vi "Render.vi"(8 "error in (no error)":errorcluster, 10 "String in":string, 11 "FencedCodeBlock in":refnum<class "FencedCodeBlock.lvclass">) -> (0 "error out":errorcluster, 2 "String out":string, 3 "FencedCodeBlock out":refnum<class "FencedCodeBlock.lvclass">)   [LabVIEW 2021, in "LvMarkdown.lvlib" / "FencedCodeBlock.lvclass"]
uses:
  FencedCodeBlock.lvclass
  C:/GitHub/LvMarkdown/src/LvMarkdown/Markdown.lvclass
  FencedCodeBlock.lvclass/FencedCodeBlock.ctl
  GetLanguage.vi
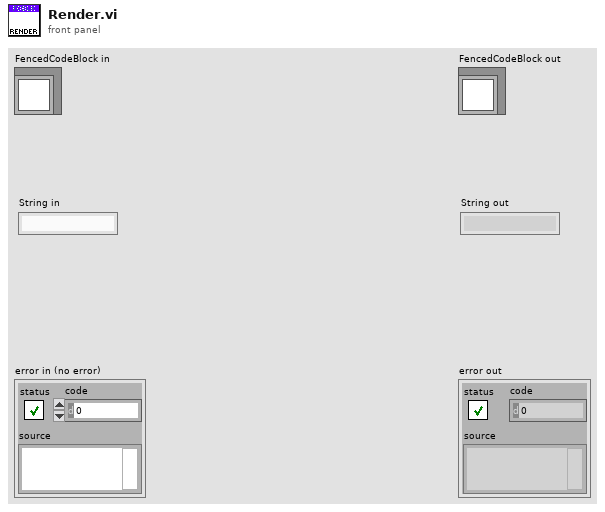
[diagram p1: front panel]
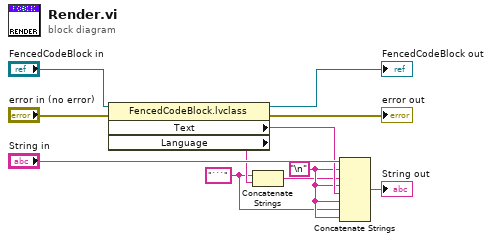
[diagram p0: block diagram]
diagram:
  w1 = "```" ("string")
  w9 = "\n"
  n1 = property class="FencedCodeBlock.lvclass"(reference="FencedCodeBlock in", error in="error in (no error)") -> (reference out=→"FencedCodeBlock out":refnum<class "FencedCodeBlock.lvclass">, error out=→"error out":errorcluster, "Text"=w10:string, "Language"=w3:string)
  n2 = Concatenate Strings(w1, w3) -> (w2:string)
  n3 = Concatenate Strings("String in", w9, w2, w9, w10, w9, w1, w9) -> (→"String out":string)
